vi "asdk Set Vector.vi"(8 "error in (no error)":errorcluster, 9 "value":dbl[](array[numeric]), 10 "command":string, 11 "pDm":u32) -> (0 "error out":errorcluster, 3 "pDm out":u32)   [LabVIEW 2010, in "ASDK.lvlib"]
doc: "ASDK_API COMPL_STAT asdkSet( asdkDM *pDm, CStrConst command, Scalar value );"
uses:
  ASDK.lvlib
  ASDK.dll
panel:
  in  "size":i32
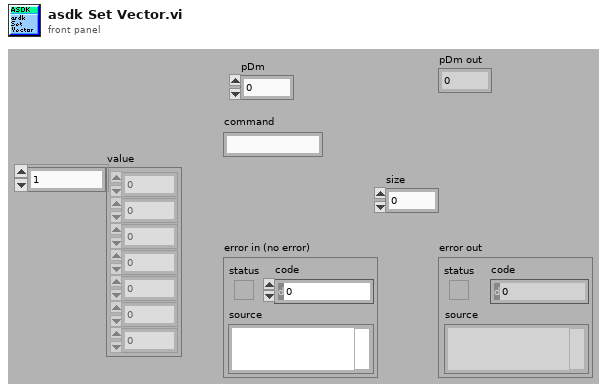
[diagram p1: front panel]
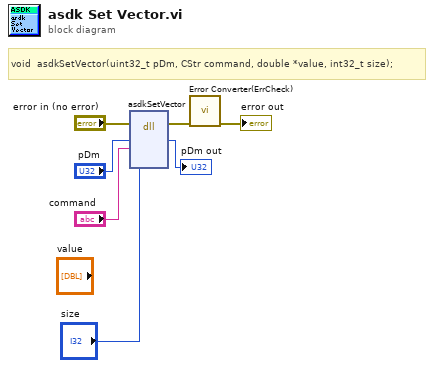
[diagram p0: block diagram]
diagram:
  # "void  asdkSetVector(uint32_t pDm, CStr command, double *value, int32_t size);"
  n1 = dll-call lib="ASDK.*" fn="asdkSetVector"(error in="error in (no error)", "pDm"="pDm", "command"="command", "size"="size") -> (error out=w3:errorcluster, "pDm"=→"pDm out":u32)  [unwired: 7 in, 1 out]
  n2 = call "Error Converter(ErrCheck).vi"("error in (no error)"=w3) -> ("error out"=→"error out":errorcluster)  [unwired: 10 in]
